vi "Measurement Logic.vi"(8 "error in":errorcluster, 10 "measurement configuration":T3={"relay name"="", "channel"="", "relay action"=21} {"relay action" items=["Open Relay"=20, "Close Relay"=21]}, 11 "measure call context in":refnum<class "Measure Call Context.lvclass">) -> (0 "error out":errorcluster, 2 "measurement results":T1={"initial relay position"=10, "final relay position"=10} {"final relay position" items=["Open"=10, "Closed"=11]; "initial relay position" items=["Open"=10, "Closed"=11]}, 3 "measure call context out":refnum<class "Measure Call Context.lvclass">)   [LabVIEW 2021, in "NI-Switch Control Relay.lvlib"]
uses:
  NI-Switch Control Relay.lvlib
  Source/Sessions/niSwitch/Session Management niSwitch.lvlib
  <vilib>/Plug-In SDKs/Measurements/Measure Call Context/Measure Call Context.lvclass
  <vilib>/Plug-In SDKs/Clients/Session Management V1/Session Reservation/Session Reservation.lvclass
  <vilib>/Plug-In SDKs/Measurements/Measure Call Context/Reserve Sessions - 1Pin.vi
  Source/Sessions/niSwitch/Initialize Sessions - 1Sess.vi
  <instrlib>/niSwitch/niSwitch.llb/niSwitch Topologies.ctl
  Measurement Configuration.ctl
  Measurement Results.ctl
  <instrlib>/niSwitch/niSwitch.llb/niSwitch Relay Action.ctl
  <instrlib>/niSwitch/niSwitch.llb/niSwitch Relay Position.ctl
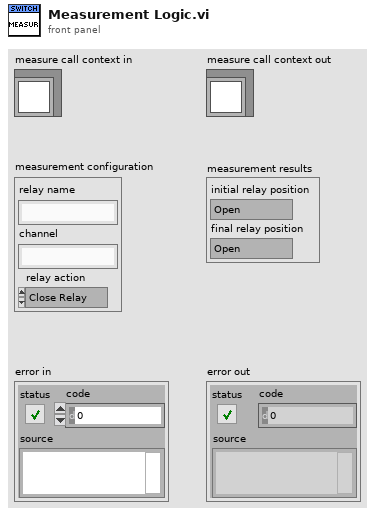
[diagram p1: front panel]
types:
  T1 = typedef "NI-Switch Control Relay.lvlib/Measurement Results.ctl" = cluster{"initial relay position":T2, "final relay position":T2}
  T2 = typedef "niSwitch Relay Position.ctl" = i32
  T3 = typedef "NI-Switch Control Relay.lvlib/Measurement Configuration.ctl" = cluster{"relay name":string, "channel":string, "relay action":T4}
  T4 = typedef "niSwitch Relay Action.ctl" = i32
  T5 = typedef "niSwitch Topologies.ctl" = string
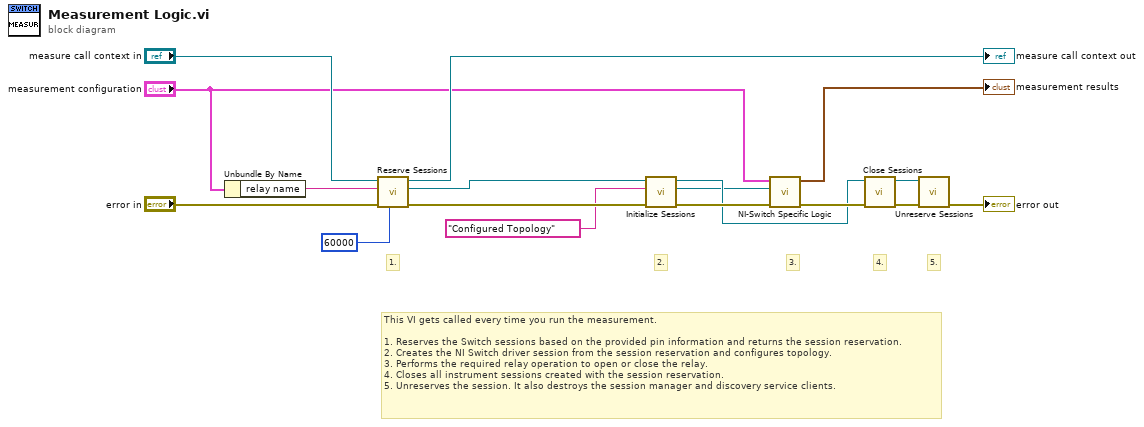
[diagram p0: block diagram]
diagram:
  # "5."
  # "4."
  # "3."
  # "2."
  # "1."
  # "This VI gets called every time you run the measurement.\n\n1. Reserves the Switch sessions based on the provided pin information and returns the session reservation.\n2. Creates the NI Switch driver session from the session reservation and configures topology. \n3. Performs the required relay operation to open or close the relay.\n4. Closes all instrument sessions created with the session reservation.\n5. Unreserves the session. It also destroys the session manager and discovery service clients."
  n1 = Unbundle By Name("measurement configuration") -> ("relay name"=w3:string)
  n2 = call-poly <vilib>:"Reserve Sessions.vi"("timeout (ms)"=60000, "error in"="error in", "pin or relay name"=w3, "measurement context in"="measure call context in") -> ("error out"=w16:errorcluster, "session reservation out"=w11:refnum<class "Session Reservation.lvclass">, "measurement context out"=→"measure call context out":refnum<class "Measure Call Context.lvclass">)  [unwired: 5 in]
  n3 = call-poly "Initialize Sessions.vi"("error in"=w16, "topology name"=T5 "Configured Topology", "session reservation in"=w11) -> ("error out"=w15:errorcluster, "session"=w9:refnum<class "Session Factory.lvclass">, "session reservation out"=w10:refnum<class "Session Reservation.lvclass">)  [unwired: 5 in, 1 out]
  n4 = call "NI-Switch Specific Logic.vi"("error in"=w15, "session factory in"=w9, "measurement configuration"="measurement configuration") -> ("error out"=w14:errorcluster, "measurement results"=→"measurement results":T1)  [unwired: 7 in]
  n5 = call <vilib>:"Close Sessions.vi"("error in"=w14, "session reservation in"=w10) -> ("error out"=w5:errorcluster, "session reservation out"=w6:refnum<class "Session Reservation.lvclass">)  [unwired: 8 in]
  n6 = call <vilib>:"Unreserve Sessions.vi"("error in"=w5, "session reservation in"=w6) -> ("error out"=→"error out":errorcluster)  [unwired: 9 in]
